vi "piezoSimple.vi"() -> ()   [LabVIEW 2017]
uses:
  globalUtilities.vi
panel:
  in  "piezo1":dbl=100.0 min=0.0 max=200.0 format="%.2g"
  in  "stop 2":bool
  in  "stop motion":bool
  in  "scan":bool
  in  "stop":bool
  in  "input":dbl format="%.2f"
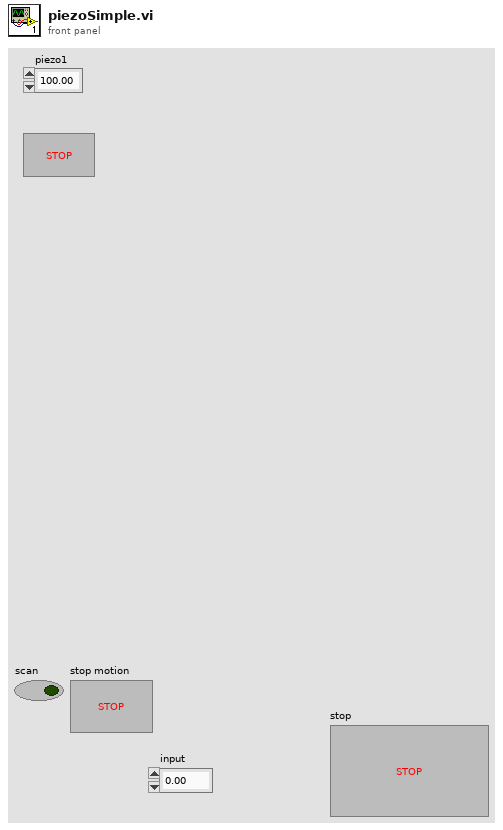
[diagram p1: front panel]
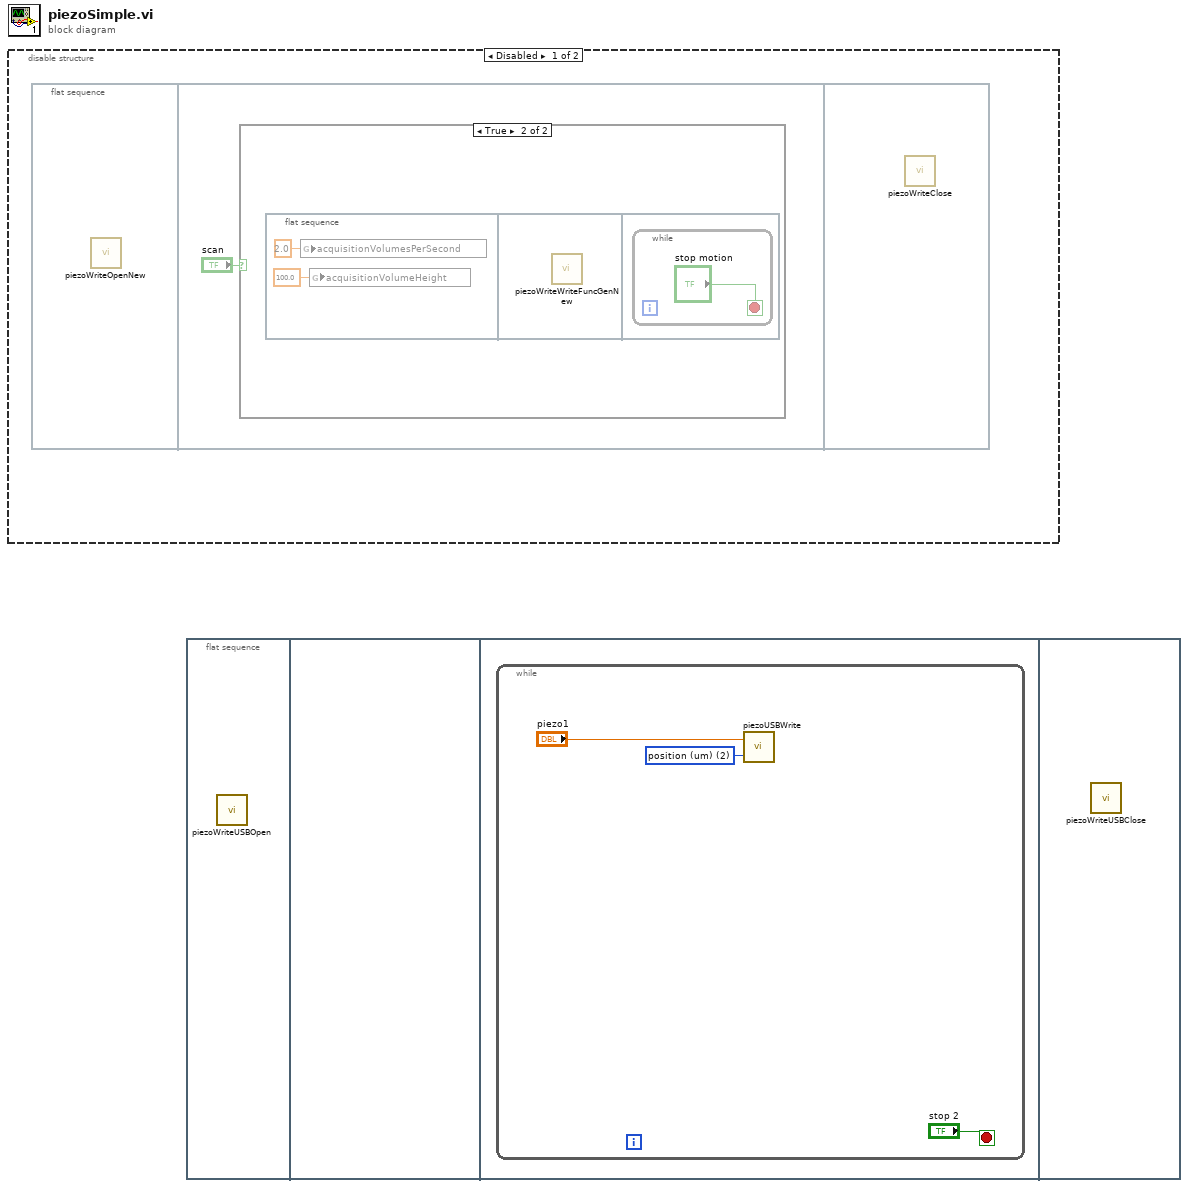
[diagram p0: block diagram]
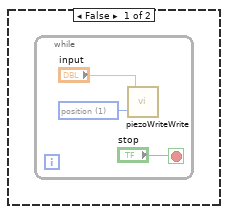
[diagram p2: hidden frame]
diagram:
  n1 = disable-structure shown="Disabled" {
    frame Disabled {
      n2 = flat-sequence {
        frame #0 {
          n3 = call "piezoWriteOpenNew.vi"() -> ()  [unwired: 2 in]
        }
        frame #1 {
          n4 = case shown="True" "scan" {
            frame False {
              n5 = while {
                stop <- "stop" stop-if-true
                w4 = u16 1 items=["fractional", "position", "voltage"] ("mode")
                n6 = call "piezoWriteWrite.vi"("mode"=w4, "input"="input") -> ()  [unwired: 1 in]
              }
            }
            frame True {
              n7 = flat-sequence {
                frame #0 {
                  n8 = global write "globalUtilities.vi" "acquisitionVolumesPerSecond"(2.0 ("acquisitionVolumesPerSecond")) -> ()
                  n9 = global write "globalUtilities.vi" "acquisitionVolumeHeight"(100.0 ("acquisitionVolumeHeight")) -> ()
                }
                frame #1 {
                  n10 = call "piezoWriteWriteFuncGenNew.vi"() -> ()  [unwired: 12 in]
                }
                frame #2 {
                  n11 = while {
                    stop <- "stop motion" stop-if-true
                  }
                }
              }
            }
          }
        }
        frame #2 {
          n12 = call "piezoWriteClose.vi"() -> ()  [unwired: 1 in]
        }
      }
    }
    frame Enabled {
    }
  }
  n13 = flat-sequence {
    frame #0 {
      n14 = call "piezoWriteUSBOpen.vi"() -> ()  [unwired: 12 in]
    }
    frame #1 {
    }
    frame #2 {
      n15 = while {
        stop <- "stop 2" stop-if-true
        w8 = u16 2 items=["fractional", "voltage (V)", "position (um)"] ("mode")
        n16 = call "piezoUSBWrite.vi"("mode"=w8, "position"="piezo1") -> ()  [unwired: 1 in]
      }
    }
    frame #3 {
      n17 = call "piezoWriteUSBClose.vi"() -> ()  [unwired: 12 in]
    }
  }
